vi "Connection Mode Generation CTS Received.vi"(0 "Connection Cluster":T3 {"Packets"."Identifier" format="%08x"}, 5 "CAN frame":T1 {"payload" format="%x"; "timestamp" format="%<%.7X\n%x>T"; "type" items=["CAN Data"=0, "CAN Remote"=1, "CAN Bus Error"=2, "J1939 Data"=192, "Delay"=224, "Log Trigger"=225, "Start Trigger"=226]; "identifier" format="%x"}, 11 "error in (no error)":errorcluster) -> (4 "Connection Cluster Out":T3 {"Packets"."Identifier" format="%08x"}, 15 "error out":errorcluster)   [LabVIEW 2013, in "J1939.lvlib"]
uses:
  J1939.lvlib
  Connection Mode Generation Connection Cluster.ctl
  API Types/CAN Outgoing Message Cluster.ctl
  <vilib>/xnet/xnet.llb/XNET Frame CAN.ctl
  <vilib>/xnet/xnet.llb/XNET Frame Type CAN.ctl
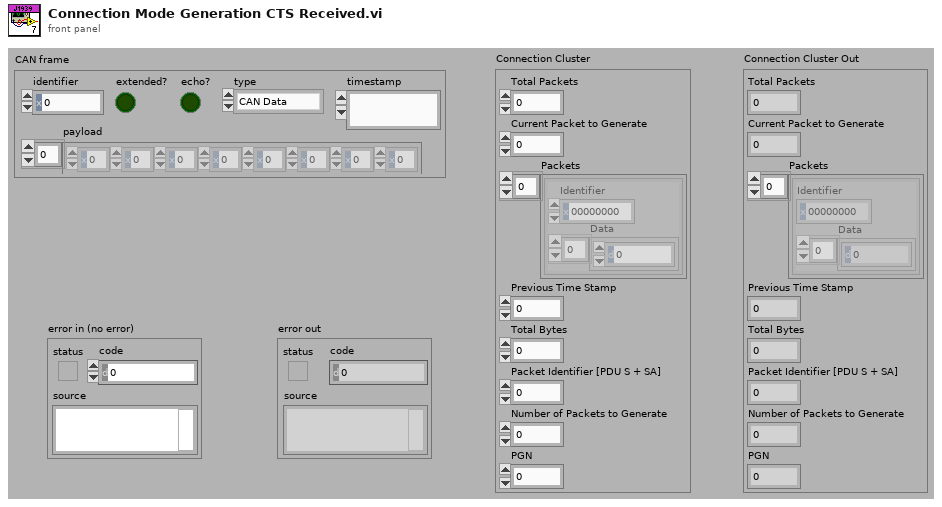
[diagram p1: front panel]
types:
  T1 = typedef "XNET Frame CAN.ctl" = cluster{"timestamp":timestamp, "payload":u8[], "identifier":u32, "type":T2, "extended?":bool, "echo?":bool}
  T2 = typedef "XNET Frame Type CAN.ctl" = u8
  T3 = typedef "J1939.lvlib/Connection Mode Generation Connection Cluster.ctl" = cluster{"Total Packets":u8, "Current Packet to Generate":u8, "Packets":T4[], "Previous Time Stamp":u32, "Total Bytes":u16, "Packet Identifier [PDU S + SA]":u16, "Number of Packets to Generate":u8, "PGN":u32}
  T4 = typedef "J1939.lvlib/CAN Outgoing Message Cluster.ctl" = cluster{"Identifier":u32, "Data":u8[]}
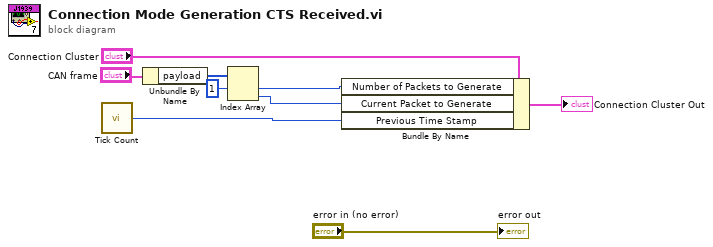
[diagram p0: block diagram]
diagram:
  n1 = call "Tick Count"() -> ("Tick Count(mSec)"=w2:u32)
  n2 = Unbundle By Name("CAN frame") -> ("payload"=w9:u8[])
  n3 = Index Array(array=w9, index #1=1 ("index")) -> (element #1=w7:u8, element #2=w6:u8)  [unwired: 1 in]
  n4 = Bundle By Name(cluster="Connection Cluster", "Number of Packets to Generate"=w7, "Current Packet to Generate"=w6, "Previous Time Stamp"=w2) -> (→"Connection Cluster Out":T3)
  "error out" <- "error in (no error)"
